vi "Initialize.vi"(7 "prompt? (F)":bool, 8 "error in":errorcluster, 9 "password":string, 10 "userID":string, 11 "connection information":path) -> (0 "error out":errorcluster, 3 "connection reference":T1)   [LabVIEW 2023, in "SQL Database.lvlib"]
uses:
  SQL Database.lvlib
  <vilib>/addons/database/NI_Database_API.lvlib
  <vilib>/addons/database/Connection.llb/DB Tools Open Connec (Path).vi
  <vilib>/addons/database/Connection.llb/Conn ObjectReference.ctl
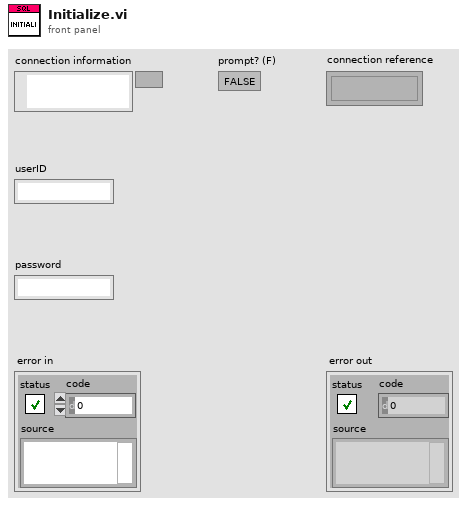
[diagram p1: front panel]
types:
  T1 = typedef "NI_Database_API.lvlib/Conn ObjectReference.ctl" = refnum<k1>
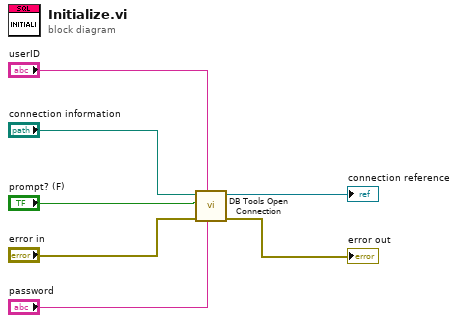
[diagram p0: block diagram]
diagram:
  n1 = call-poly <vilib>:"DB Tools Open Connection.vi"("password"="password", "userID"="userID", "error in (no error)"="error in", "prompt? (F)"="prompt? (F)", "connection information"="connection information") -> ("error out"=→"error out":errorcluster, "connection reference"=→"connection reference":T1)  [unwired: 3 in]
